vi "HardwareInit.vi"(8 "Error/Flow In":errorcluster) -> (0 "error out":errorcluster)   [LabVIEW 2018]
panel:
  in  "Controllers Port":tag="A/I2C"
  in  "Servo Controller ID":u8=3 min=1 max=4
  in  "Motor Controller 2 ID":u8=2 min=1 max=4
  in  "Motor Controller 1 ID":u8=1 min=1 max=4
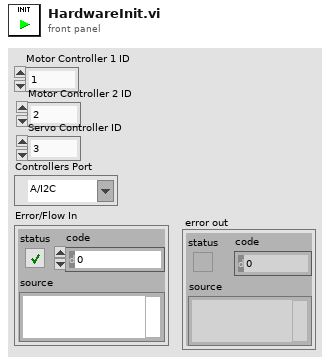
[diagram p1: front panel]
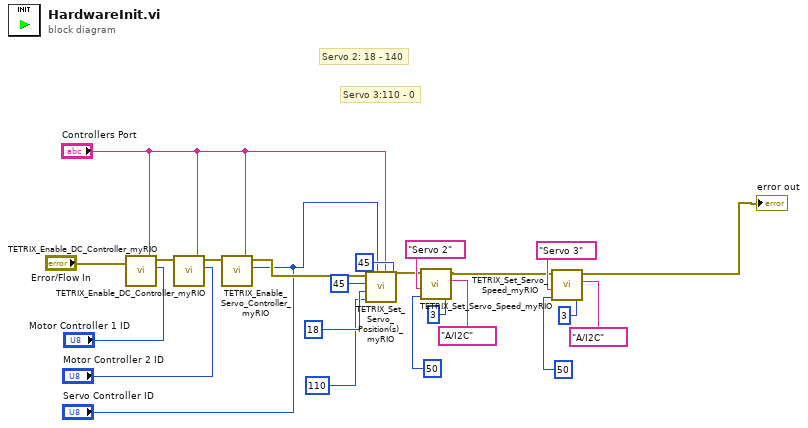
[diagram p0: block diagram]
diagram:
  # "Servo 3:110 - 0"
  # "Servo 2: 18 - 140"
  n1 = call <vilib>:"TETRIX_Enable_DC_Controller_myRIO.vi"("myRIO MXP Port A/B"="Controllers Port", "Controller ID#  (I2C Address)"="Motor Controller 1 ID", "Error/Flow In"="Error/Flow In") -> ("Error/Flow Out"=w22:errorcluster)  [unwired: 4 in]
  n2 = call <vilib>:"TETRIX_Enable_DC_Controller_myRIO.vi"("myRIO MXP Port A/B"="Controllers Port", "Controller ID#  (I2C Address)"="Motor Controller 2 ID", "Error/Flow In"=w22) -> ("Error/Flow Out"=w23:errorcluster)  [unwired: 4 in]
  n3 = call <vilib>:"TETRIX_Enable_Servo_Controller_myRIO.vi"("myRIO MXP Port A/B"="Controllers Port", "Controller ID#  (I2C Address)"="Servo Controller ID", "Error/Flow In"=w23) -> ("Error/Flow Out"=w18:errorcluster)  [unwired: 4 in]
  n4 = call <vilib>:"TETRIX_Set_Servo_Position(s)_myRIO.vi"("Servo 4 Position (0 - 180 degrees)"=u8 45, "myRIO MXP Port A/B"="Controllers Port", "Controller ID#  (I2C Address)"="Servo Controller ID", "Servo 3 Position (0 - 180 degrees)"=u8 110, "Servo 2 Position (0 - 180 degrees)"=u8 18, "Servo 1 Position (0 - 180 degrees)"=u8 45, "Error/Flow In"=w18) -> ("Error/Flow Out"=w7:errorcluster)  [unwired: 2 in]
  n5 = call <vilib>:"TETRIX_Set_Servo_Speed_myRIO.vi"("myRIO MXP Port A/B"=tag "A/I2C", "Set Servo Speed (0 - 100 percent)"=u8 50, "Select Channel"="Servo 2", "Controller ID#  (I2C Address)"=u8 3, "Error/Flow In"=w7) -> ("Error/Flow Out"=w2:errorcluster)  [unwired: 2 in]
  n6 = call <vilib>:"TETRIX_Set_Servo_Speed_myRIO.vi"("myRIO MXP Port A/B"=tag "A/I2C", "Set Servo Speed (0 - 100 percent)"=u8 50, "Select Channel"="Servo 3", "Controller ID#  (I2C Address)"=u8 3, "Error/Flow In"=w2) -> ("Error/Flow Out"=→"error out":errorcluster)  [unwired: 2 in]
